vi "Global_ACT Write_Data Out.vi"() -> ()   [LabVIEW 2017]
uses:
  TypeDef/CLUSTER_Drive_HW_SRX_Status.ctl
  _SHARE ALL/RoboRio Share All/SRX Share All/TypeDefs SRX/Cluster_SRX_Common Runtime Data.ctl
  _SHARE ALL/RoboRio Share All/SRX Share All/TypeDefs SRX/Cluster_SRX_Error Calculations.ctl
  _SHARE ALL/RoboRio Share All/SRX Share All/TypeDefs SRX/Cluster_SRX_Voltage Out Data.ctl
  _SHARE ALL/RoboRio Share All/SRX Share All/TypeDefs SRX/Cluster_SRX_Sensor Out Data.ctl
panel:
  in  "WC_Drive_HW_SRX_Status":T1 {"Left"."Temp" format="%.1f"; "Left"."Voltage"."Bus" format="%.3f"; "Left"."Voltage"."Output" format="%.3f"; "Left"."Voltage"."Percent" format="%.3f"; "Left"."Current" format="%.2f"; "Right"."Temp" format="%.1f"; "Right"."Voltage"."Bus" format="%.3f"; "Right"."Voltage"."Output" format="%.3f"; "Right"."Voltage"."Percent" format="%.3f"; "Right"."Current" format="%.2f"}
  # "The Names of the Data items in the Global Variable MUST describe who the Single Writer is\nNaming Convention of all Data Items is:   Lib Name_Loop Name (SM or SEN or ACT)_Data Name\nExample   Drive_ACT_X axis;  GameController_SEN_JoystickLeft;  Hopper_SM_AgitatorSpeed"
  # "C"
  # "Units"
  # "C"
  # "Units"
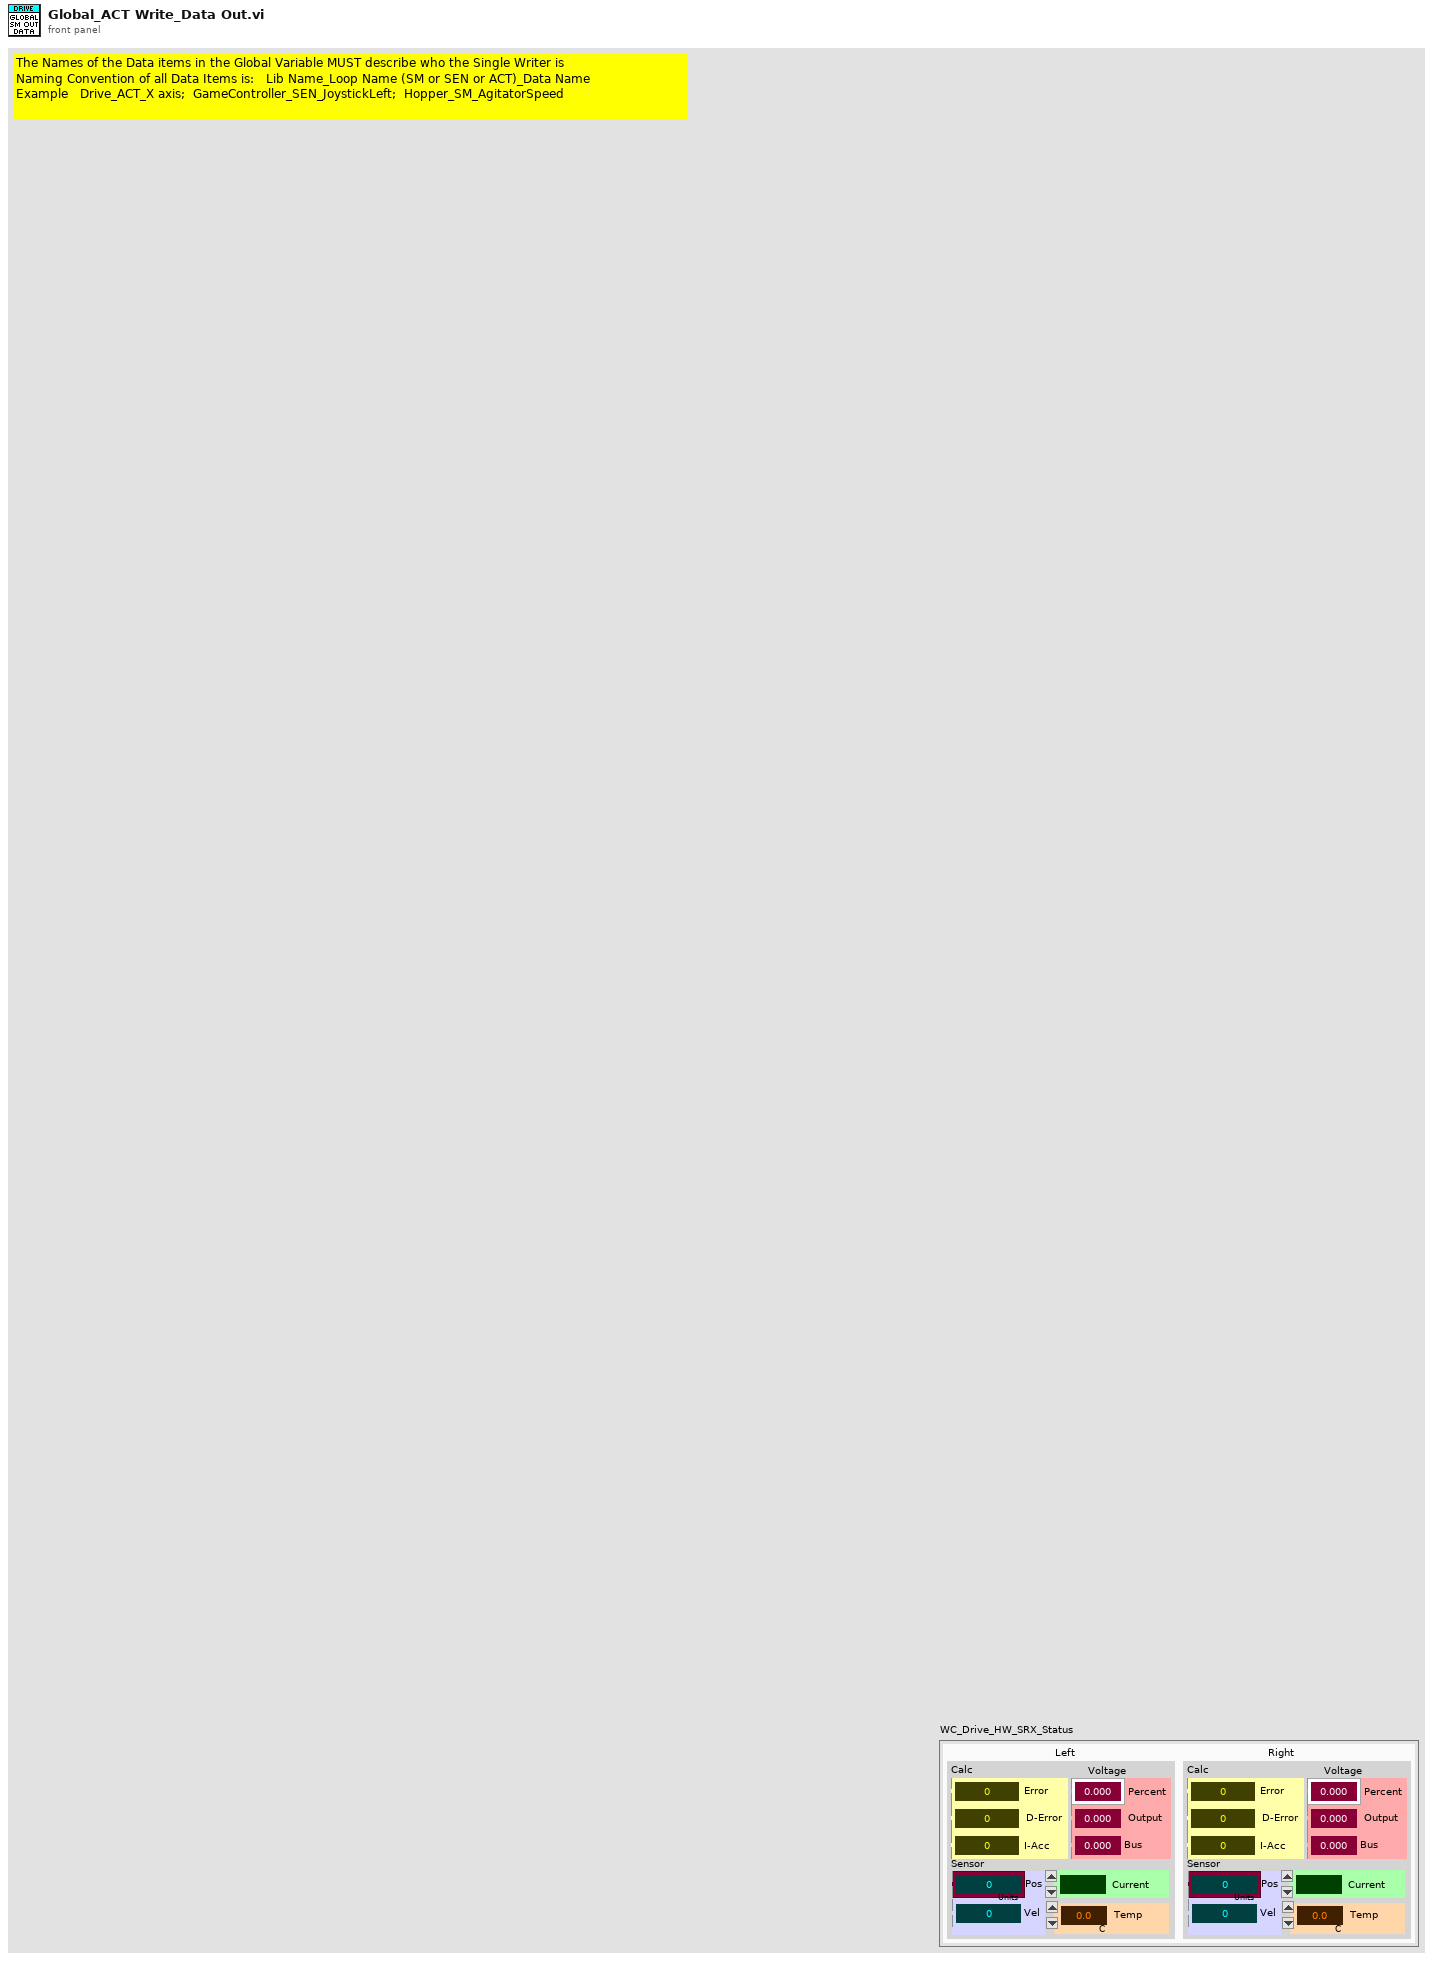
[diagram p1: front panel]
types:
  T1 = typedef "CLUSTER_Drive_HW_SRX_Status.ctl" = cluster{"Left":T2, "Right":T2}
  T2 = typedef "Cluster_SRX_Common Runtime Data.ctl" = cluster{"Calc":T3, "Voltage ":T4, "Sensor":T5, "Current":dbl, "Temp":dbl}
  T3 = typedef "Cluster_SRX_Error Calculations.ctl" = cluster{"Error":i32, "D-Error":dbl, "I-Acc":dbl}
  T4 = typedef "Cluster_SRX_Voltage Out Data.ctl" = cluster{"Percent":dbl, "Output":dbl, "Bus":dbl}
  T5 = typedef "Cluster_SRX_Sensor Out Data.ctl" = cluster{"Pos":i32, "Vel":i32}
diagram:
